vi "Shut Down Device.vi"(8 "error in (no error)":errorcluster, 11 "Microsync in":refnum<class "Microsync.lvclass">) -> (0 "error out":errorcluster, 3 "Microsync out":refnum<class "Microsync.lvclass">)   [LabVIEW 2023, in "Microsync.lvlib" / "Microsync.lvclass"]
uses:
  Microsync.lvclass
  Microsync.lvclass/Microsync.ctl
  Sync Device/Sync Device.lvclass
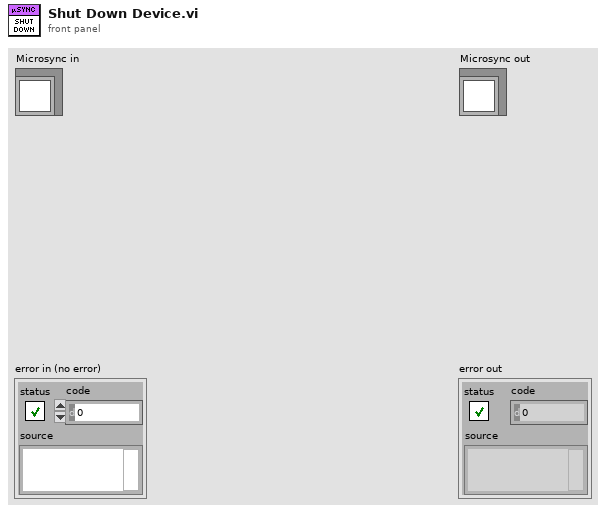
[diagram p1: front panel]
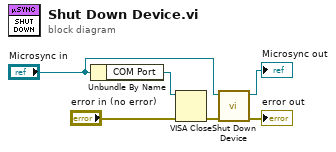
[diagram p0: block diagram]
diagram:
  n1 = Unbundle By Name("Microsync in") -> ("COM Port"=w1:refnum<visa-resource-name>)
  n2 = VISA Close(VISA resource name=w1, error in (no error)="error in (no error)") -> (error out=w4:errorcluster)
  n3 = call-parent "Shut Down Device.vi"("error in (no error)"=w4, "Device in"="Microsync in") -> ("error out"=→"error out":errorcluster, "Device out"=→"Microsync out":refnum<class "Microsync.lvclass">)  [unwired: 8 in]
